vi "Vars.vi"(2 "name or relative path":string, 3 "Path":path) -> (0 "output":T2, 1 "input":T1)   [LabVIEW 2019]
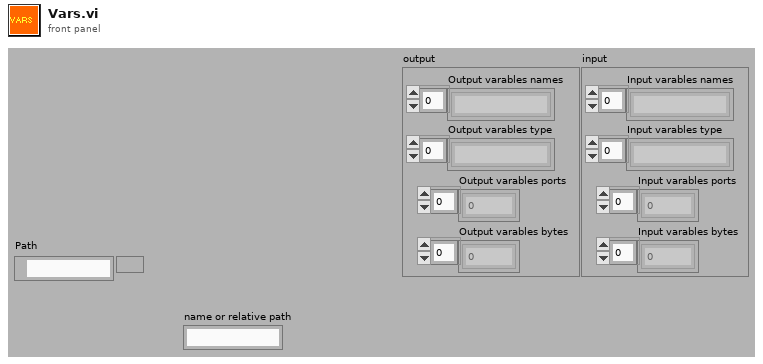
[diagram p1: front panel]
types:
  T1 = cluster{"Input varables names":string[], "Input varables type":string[], "Input varables ports":i32[], "Input varables bytes":i32[]}
  T2 = cluster{"Output varables names":string[], "Output varables type":string[], "Output varables ports":i32[], "Output varables bytes":i32[]}
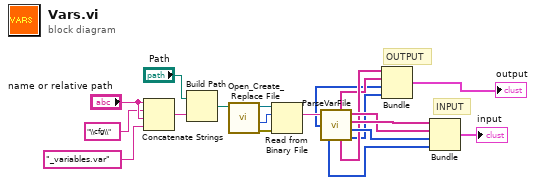
[diagram p0: block diagram]
diagram:
  # "OUTPUT"
  # "INPUT"
  n1 = Concatenate Strings("name or relative path", "\\cfg\\" ("string"), "name or relative path", "_variables.var" ("name or relative path")) -> (w13:string)
  n2 = Build Path(base path="Path", name or relative path=w13) -> (appended path=w15:path)
  n3 = call <vilib>:"Open_Create_Replace File.vi"("file path"=w15) -> ("error out"=w16:errorcluster, "file size (bytes)"=w17:i32, "refnum"=w18:refnum<file>)  [unwired: 7 in, 1 out]
  n4 = Read from Binary File(8:w16, 10:w17, 11:w18) -> (2:w11:string)  [unwired: 3 in, 3 out]
  n5 = call "ParseVarFile.vi"("data"=w11) -> ("Output varables bytes"=w3:i32[], "Output varables names"=w6:string[], "Input varables ports"=w8:i32[], "Input varables names"=w10:string[], "Output varables type"=w5:string[], "Input varables type"=w9:string[], "Input varables bytes"=w7:i32[], "Output varables ports"=w4:i32[])
  n6 = Bundle("Output varables names"=w6, "Output varables type"=w5, "Output varables ports"=w4, "Output varables bytes"=w3) -> (→"output":T2)  [unwired: 1 in]
  n7 = Bundle("Input varables names"=w10, "Input varables type"=w9, "Input varables ports"=w8, "Input varables bytes"=w7) -> (→"input":T1)  [unwired: 1 in]
